vi "ClearNoise Log.vi"(7 "ACQ full DATA file path":path caption="File path", 8 "Log it":i32, 9 "ClearNoise vars":T1={"Waiting time X"=0, "ClearNoise ACQits"=4, "Threshold Z"=1000, "HVit Refnum"=refnum, "ACQit Refnum"=refnum} {"ClearNoise ACQits" min=1 step=1}, 10 "Killing list B":T2(array[cluster]) {"ChipID" format="%.0x"}, 11 "Killing list A":T2(array[cluster]) {"ChipID" format="%.0x"}) -> ()   [LabVIEW 2015, in "VIPM2.lvlib"]
uses:
  VIPM2.lvlib
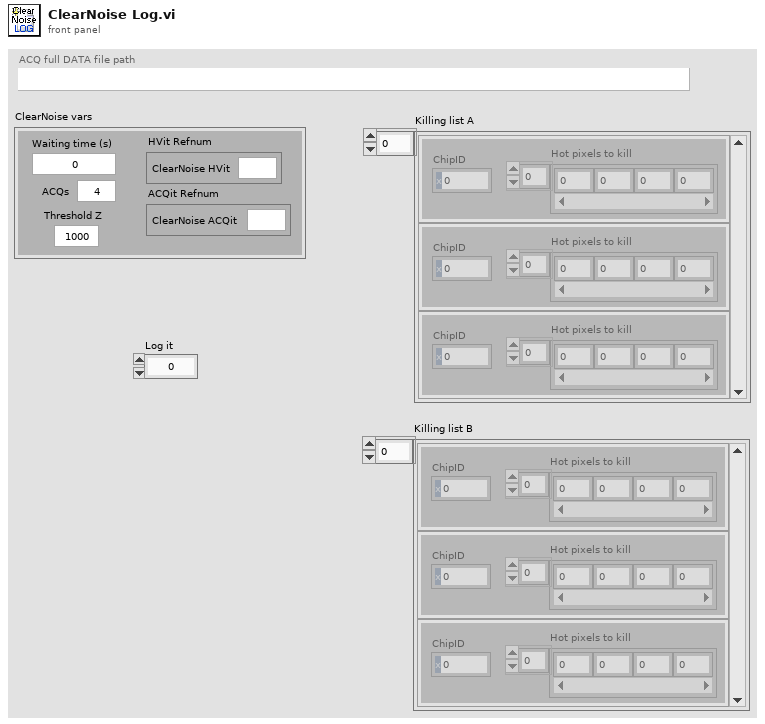
[diagram p1: front panel]
types:
  T1 = cluster{"Waiting time X":u32, "ClearNoise ACQits":i32, "Threshold Z":u32, "HVit Refnum":refnum<vi>, "ACQit Refnum":refnum<vi>}
  T2 = cluster{"ChipID":u16, "Hot pixels to kill":u8[]}[]
  T3 = enum16{"open", "replace", "create", "open or create", "replace or create", "replace or create with confirmation"}
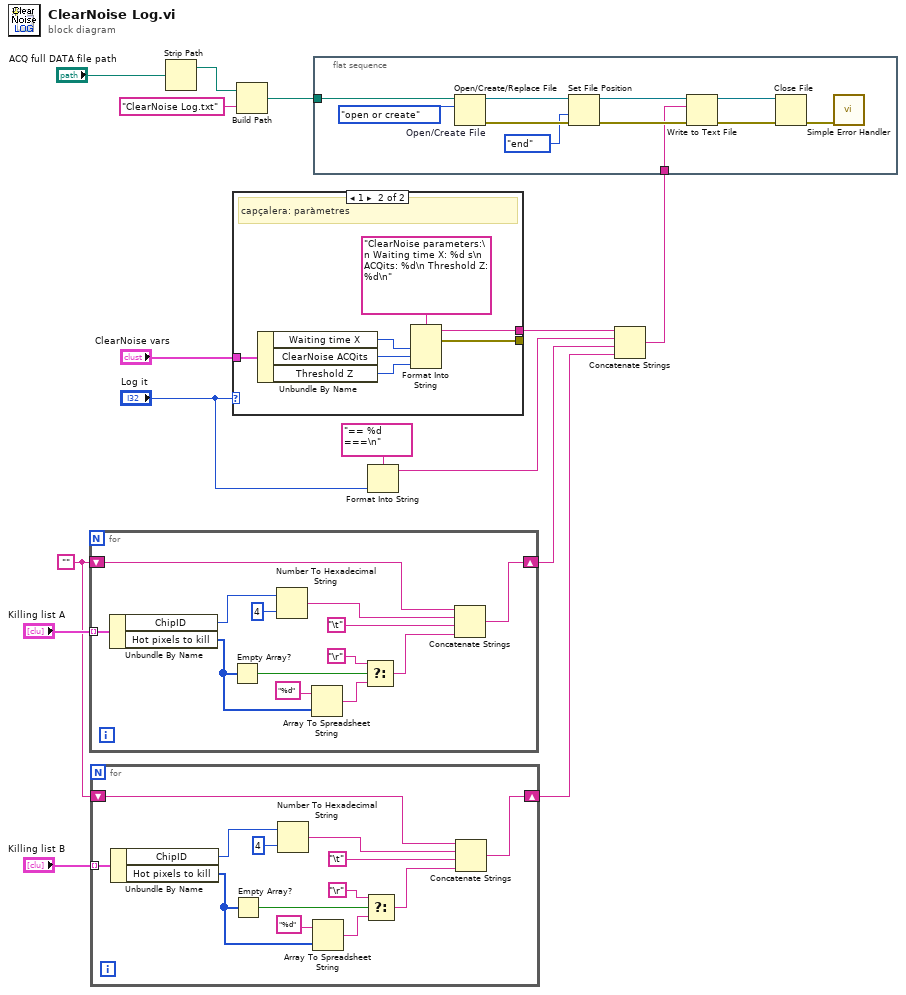
[diagram p0: block diagram]
diagram:
  w3 = ""
  n1 = for {
    tunnel: "Killing list A" -> [w28] mode=indexing
    shift-right: [w23] -> w5
    shift-left: w3 -> [w24]
    n2 = Unbundle By Name(w28) -> ("ChipID"=w27:u16, "Hot pixels to kill"=w21:u8[])
    n3 = Empty Array?(array=w21) -> (empty?=w18:bool)
    n4 = Number To Hexadecimal String(1:i16 4 ("width (-)"), 2:w27) -> (0:w25:string)
    n5 = Array To Spreadsheet String(array=w21, 3:"%d" ("format string")) -> (spreadsheet string=w19:string)  [unwired: 1 in]
    n6 = Select(t="\r", s=w18, f=w19) -> (s? t:f=w16:string)
    n7 = Concatenate Strings "Concatenate Strings"(w24, w25, "\t", w16) -> (w23:string)
  }
  n8 = for {
    tunnel: "Killing list B" -> [w41] mode=indexing
    shift-right: [w36] -> w1
    shift-left: w3 -> [w37]
    n9 = Unbundle By Name(w41) -> ("ChipID"=w40:u16, "Hot pixels to kill"=w34:u8[])
    n10 = Empty Array?(array=w34) -> (empty?=w31:bool)
    n11 = Number To Hexadecimal String(1:i16 4 ("width (-)"), 2:w40) -> (0:w38:string)
    n12 = Array To Spreadsheet String(array=w34, 3:"%d" ("format string")) -> (spreadsheet string=w32:string)  [unwired: 1 in]
    n13 = Select(t="\r", s=w31, f=w32) -> (s? t:f=w29:string)
    n14 = Concatenate Strings "Concatenate Strings"(w37, w38, "\t", w29) -> (w36:string)
  }
  n15 = Strip Path(path="ACQ full DATA file path") -> (stripped path=w14:path)  [unwired: 1 out]
  n16 = case shown="1" "Log it" {
    tunnel: "ClearNoise vars" -> [_ w48]
    tunnel: [_ w43] -> w8
    tunnel: [_ w42] -> _
    frame Default {
    }
    frame 1 {
      # "capçalera: paràmetres"
      n17 = Unbundle By Name(w48) -> ("Waiting time X"=w45:u32, "ClearNoise ACQits"=w46:i32, "Threshold Z"=w44:u32)
      n18 = Format Into String "Format Into String"(format string="ClearNoise parameters:\n Waiting time X: %d s\n ACQits: %d\n Threshold Z: %d\n", w45, w46, w44) -> (resulting string=w43:string, error out=w42:errorcluster)  [unwired: 2 in]
    }
  }
  n19 = Build Path(base path=w14, name or relative path="ClearNoise Log.txt") -> (appended path=w12:path)
  n20 = flat-sequence {
    tunnel: w12 -> [w58]
    tunnel: w4 -> [w49]
    frame #0 {
      n21 = Open/Create/Replace File "Open/Create File"(file path (use dialog)=w58, operation (0:open)=T3."open or create") -> (refnum out=w57:refnum<file>, error out=w56:errorcluster)  [unwired: 4 in, 1 out]
      n22 = Set File Position(refnum=w57, from (0:start)=enum16{"start", "end", "current"}."end", error in=w56) -> (refnum out=w54:refnum<file>, error out=w53:errorcluster)  [unwired: 1 in]
      n23 = Write to Text File(file (use dialog)=w54, text=w49, error in=w53) -> (refnum out=w52:refnum<file>, error out=w51:errorcluster)  [unwired: 1 in, 1 out]
      n24 = Close File(refnum=w52, error in=w51) -> (error out=w50:errorcluster)  [unwired: 1 out]
      n25 = call <vilib>:"Simple Error Handler.vi"("error in (no error)"=w50) -> ()  [unwired: 4 in, 5 out]
    }
  }
  n26 = Format Into String "Format Into String"(format string="== %d ===\n", "Log it") -> (resulting string=w7:string)  [unwired: 2 in, 1 out]
  n27 = Concatenate Strings "Concatenate Strings"(w8, w7, w5, w1) -> (w4:string)
